vi "aboutS0.vi"(7 "error in (no error)":errorcluster) -> (0 "error out":errorcluster)   [LabVIEW 2015, in "ESLSCDLL.lvlib"]
uses:
  ESLSCDLL.lvlib
  Globals.vi
  ESLSCDLL.dll
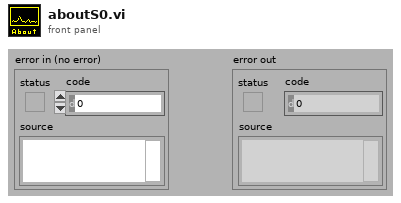
[diagram p1: front panel]
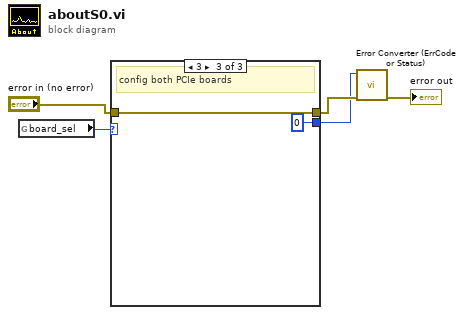
[diagram p0: block diagram]
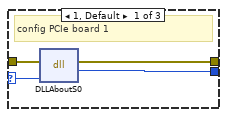
[diagram p2: hidden frame]
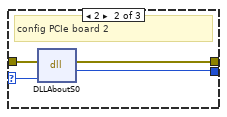
[diagram p3: hidden frame]
diagram:
  n1 = global read "Globals.vi" "board_sel"() -> (w1:u32)
  n2 = case shown="3" w1 {
    selector: w1 -> [w9 w13 _]
    tunnel: "error in (no error)" -> [w8 w12 w15]
    tunnel: [w7 w11 w15] -> w4
    tunnel: [w6 w10 0 ("es_status_codes")] -> w2
    frame 1, Default {
      # "config PCIe board 1"
      n3 = dll-call lib="C:/Users/flori/Nextcloud/Dokumente/Stresing/Windows/lv64/board.vis/ESLSCDLL.dll" fn="DLLAboutS0" ("lwlscdll.dll:DLLAboutDrv")(error in=w8, "drv"=w9) -> (error out=w7:errorcluster, "es_status_codes"=w6:i32)  [unwired: 3 in, 1 out]
    }
    frame 2 {
      # "config PCIe board 2"
      n4 = dll-call lib="C:/Users/flori/Nextcloud/Dokumente/Stresing/Windows/lv64/board.vis/ESLSCDLL.dll" fn="DLLAboutS0" ("lwlscdll.dll:DLLAboutDrv")(error in=w12, "drv"=w13) -> (error out=w11:errorcluster, "es_status_codes"=w10:i32)  [unwired: 3 in, 1 out]
    }
    frame 3 {
      # "config both PCIe boards"
    }
  }
  n5 = call "Error Converter (ErrCode or Status).vi"("error in (no error)"=w4, "error code"=w2) -> ("error out"=→"error out":errorcluster)  [unwired: 9 in]
